vi "Brow Node Factory.vi"(8 "error in (no error)":errorcluster, 11 "Brower View in":refnum<class "Brower View.lvclass">) -> (0 "error out":errorcluster, 3 "Brower View out":refnum<class "Brower View.lvclass">)   [LabVIEW 2015, in "Brower View.lvclass"]
uses:
  Brower View.lvclass
  MyTreeAPI/MyTreeAPI.lvclass
  <vilib>/ErrorRing/Error Ring.xnode
  <vilib>/Utility/error.llb/Error Cluster From Error Code.vi
  <vilib>/ActorFramework/Message Enqueuer/Message Enqueuer.lvclass
panel:
  in  "ItemTag":string
  in  "Brower Controller Q":refnum<class "Message Enqueuer.lvclass">
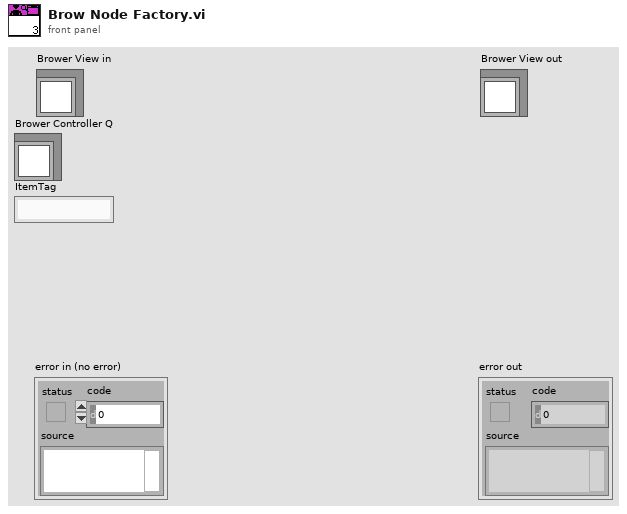
[diagram p1: front panel]
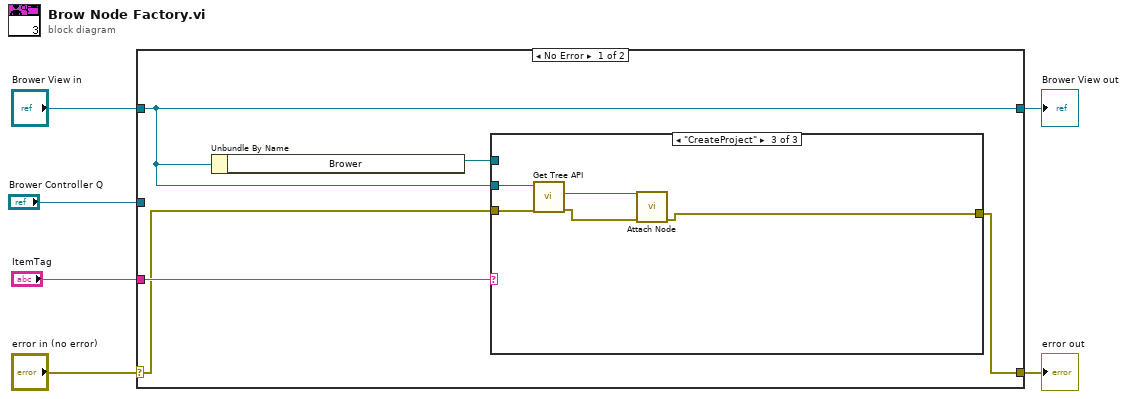
[diagram p0: block diagram]
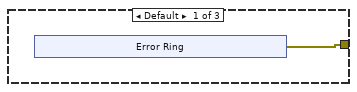
[diagram p2: hidden frame]
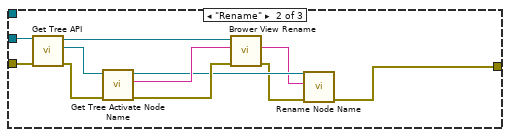
[diagram p3: hidden frame]
diagram:
  n1 = case shown="No Error" "error in (no error)" {
    selector: "error in (no error)" -> [w8 w35]
    tunnel: [w7 w35] -> w5
    tunnel: [w9 w34] -> w3
    tunnel: "Brower View in" -> [w9 w34]
    tunnel: "Brower Controller Q" -> [_ _]
    tunnel: "ItemTag" -> [w11 _]
    frame No Error {
      n2 = Unbundle By Name(w9) -> ("Brower"=w10:refnum<vi>)
      n3 = case shown="\"CreateProject\"" w11 {
        tunnel: w10 -> [_ _ _]
        tunnel: w9 -> [_ w28 w33]
        tunnel: w8 -> [_ w26 w32]
        tunnel: [w12 w18 w29] -> w7
        frame Default {
          n4 = xnode "Error Ring"() -> ("error out"=w12:errorcluster)
        }
        frame "Rename" {
          n5 = call "Get Tree API.vi"("error in (no error)"=w26, "Brower View in"=w28) -> ("error out"=w23:errorcluster, "myTree.lvclass"=w25:refnum<class "MyTreeAPI.lvclass">, "Brower View out"=w27:refnum<class "Brower View.lvclass">)  [unwired: 7 in]
          n6 = call "Get Tree Activate Node Name.vi"("error in (no error)"=w23, "MyTreeAPI in"=w25) -> ("error out"=w22:errorcluster, "Cell String"=w24:string, "MyTreeAPI out"=w21:refnum<class "MyTreeAPI.lvclass">)  [unwired: 7 in]
          n7 = call "Brower View Rename.vi"("error in (no error)"=w22, "PreviousName"=w24, "Brower View in"=w27) -> ("error out"=w19:errorcluster, "New Name Out"=w20:string)  [unwired: 6 in, 1 out]
          n8 = call "Rename Node Name.vi"("error in (no error)"=w19, "Node Tag"=w20, "TREE in"=w21) -> ("error out"=w18:errorcluster)  [unwired: 7 in, 1 out]
        }
        frame "CreateProject" {
          n9 = call "Get Tree API.vi"("error in (no error)"=w32, "Brower View in"=w33) -> ("error out"=w30:errorcluster, "myTree.lvclass"=w31:refnum<class "MyTreeAPI.lvclass">)  [unwired: 7 in, 1 out]
          n10 = call "Attach Node.vi"("TREE in"=w31, "error in (no error)"=w30) -> ("error out"=w29:errorcluster)  [unwired: 11 in, 2 out]
        }
      }
    }
    frame Error {
    }
  }
  "error out" <- w5
  "Brower View out" <- w3
